vi "FGV Graph Gas-Auswahl.vi"(6 "Aktion":T2, 10 "Graphen":T1) -> (2 "Graphen neu":T1)   [LabVIEW 2020, in "Grafik.lvlib"]
uses:
  Grafik.lvlib
  FGV Graph Gas-Auswahl Aktion.ctl
  Graphen Auswahl.ctl
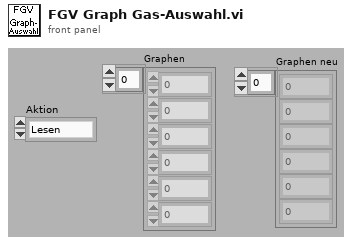
[diagram p1: front panel]
types:
  T1 = typedef "Grafik.lvlib/Graphen Auswahl.ctl" = u16[]
  T2 = typedef "Grafik.lvlib/FGV Graph Gas-Auswahl Aktion.ctl" = enum16{"Lesen", "Schreiben"}
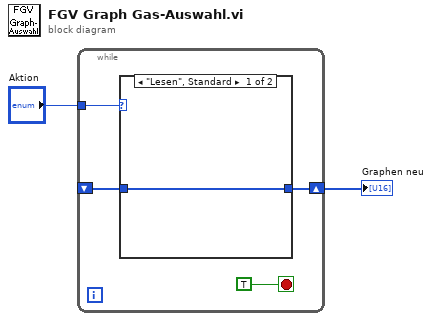
[diagram p0: block diagram]
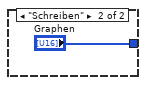
[diagram p2: hidden frame]
diagram:
  n1 = while {
    shift-right: [w4] -> w1
    shift-left: _ -> [w3]
    tunnel: "Aktion" -> [w5]
    stop <- TRUE stop-if-true
    n2 = case shown="\"Lesen\", Standard" w5 {
      tunnel: [w7 "Graphen"] -> w4
      tunnel: w3 -> [w7 _]
      frame "Lesen", Default {
      }
      frame "Schreiben" {
      }
    }
  }
  "Graphen neu" <- w1
